vi "CRYCurve averaging real-time fft.vi"(7 "Initialize (F)":bool, 8 "Exponential averaging? (F=linear)":bool, 10 "Number of averages (no change)":i32, 11 "Input curve":dbl[](array[numeric]) format="%.2f") -> (3 "Averaged curve":dbl[](array[numeric]) format="%.2f")   [LabVIEW 2013]
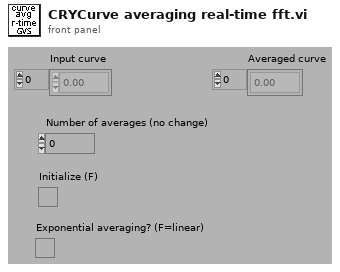
[diagram p1: front panel]
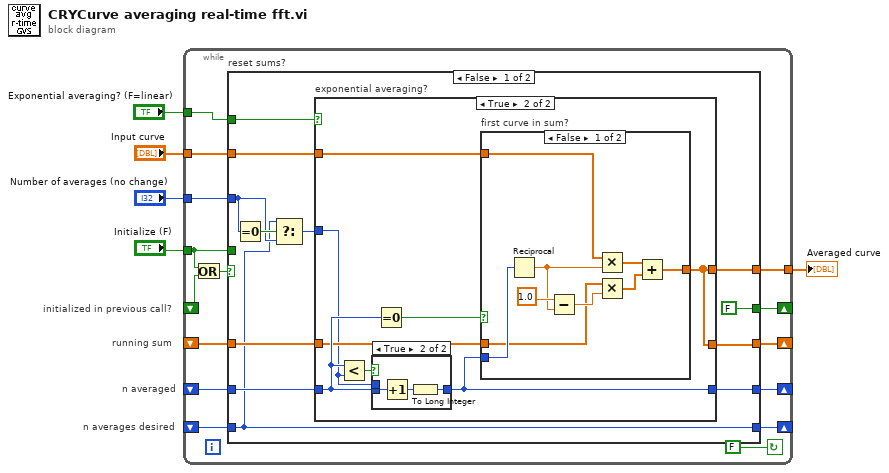
[diagram p0: block diagram]
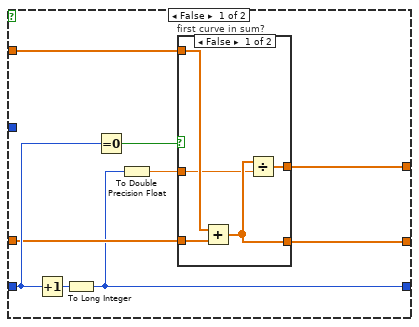
[diagram p2: hidden frame]
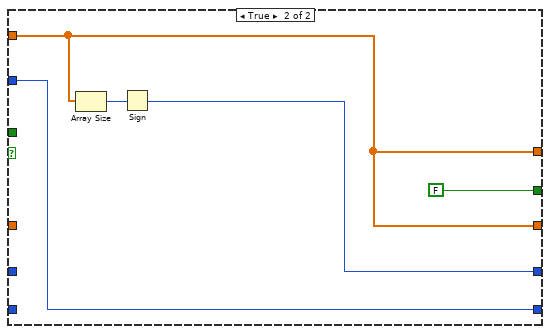
[diagram p6: hidden frame]
diagram:
  # "initialized in previous call?"
  # "n averages desired"
  # "n averaged"
  # "running sum"
  n1 = while {
    shift-left: _ -> [w8]
    shift-right: [w10] -> _
    tunnel: "Exponential averaging? (F=linear)" -> [w11]
    shift-left: _ -> [w12]
    shift-right: [w13] -> _
    tunnel: [w15] -> w2
    tunnel: "Number of averages (no change)" -> [w17]
    tunnel: "Input curve" -> [w18]
    tunnel: "Initialize (F)" -> [w9]
    shift-left: _ -> [w16]
    shift-right: [w19] -> _
    shift-left: _ -> [w14]
    shift-right: [w20] -> _
    stop <- FALSE continue-if-true
    n2 = Or(x=w9, y=w8) -> (x .or. y?=w7:bool)
    n3 = case "reset sums?" shown="False" w7 {
      tunnel: [w23 w71] -> w20
      tunnel: [w29 w70] -> w19
      tunnel: w18 -> [w31 w71]
      tunnel: w17 -> [w27 w74]
      tunnel: w16 -> [w32 _]
      tunnel: [w24 w71] -> w15
      tunnel: w14 -> [w30 _]
      tunnel: [w25 w74] -> w13
      tunnel: w12 -> [w25 _]
      tunnel: w11 -> [w22 _]
      tunnel: [FALSE ("Initialize (F)") FALSE ("Initialize (F)")] -> w10
      tunnel: w9 -> [_ _]
      frame False {
        n4 = Equal To 0?(x=w27) -> (x = 0?=w28:bool)
        n5 = Select(t=w25, s=w28, f=w27) -> (s? t:f=w26:i32)
        n6 = case "exponential averaging?" shown="True" w22 {
          tunnel: w32 -> [w40 w54]
          tunnel: w31 -> [w37 w52]
          tunnel: w30 -> [w38 w51]
          tunnel: [w34 w50] -> w29
          tunnel: [w35 w48] -> w24
          tunnel: w26 -> [_ w49]
          tunnel: [w36 w48] -> w23
          frame False {
            n7 = Increment(x=w40) -> (x+1=w41:i32)
            n8 = To Long Integer(number=w41) -> (32bit integer=w34:i32)
            n9 = Equal To 0?(x=w40) -> (x = 0?=w39:bool)
            n10 = To Double Precision Float(number=w34) -> (double precision float=w33:dbl)
            n11 = case "first curve in sum?" shown="False" w39 {
              tunnel: w38 -> [w46 _]
              tunnel: w37 -> [w45 w47]
              tunnel: [w44 w47] -> w36
              tunnel: [w43 w47] -> w35
              tunnel: w33 -> [w42 _]
              frame False {
                n12 = Add(x=w45, y=w46) -> (x+y=w44:dbl[])
                n13 = Divide(x=w44, y=w42) -> (x/y=w43:dbl[])
              }
              frame True {
              }
            }
          }
          frame True {
            n14 = Less?(x=w54, y=w49) -> (x < y?=w55:bool)
            n15 = case shown="True" w55 {
              tunnel: w54 -> [_ w69]
              tunnel: [w66 w67] -> w50
              tunnel: w49 -> [w66 _]
              frame False {
              }
              frame True {
                n16 = Increment(x=w69) -> (x+1=w68:i32)
                n17 = To Long Integer(number=w68) -> (32bit integer=w67:i32)
              }
            }
            n18 = Equal To 0?(x=w54) -> (x = 0?=w53:bool)
            n19 = case "first curve in sum?" shown="False" w53 {
              tunnel: w52 -> [w62 w65]
              tunnel: [w56 w65] -> w48
              tunnel: w51 -> [w59 _]
              tunnel: w50 -> [w64 _]
              frame False {
                n20 = Reciprocal(x=w64) -> (1/x=w61:dbl)
                n21 = Subtract(x=1.0, y=w61) -> (x-y=w60:dbl)
                n22 = Multiply(x=w62, y=w61) -> (x*y=w58:dbl[])
                n23 = Multiply(x=w59, y=w60) -> (x*y=w57:dbl[])
                n24 = Add(x=w58, y=w57) -> (x+y=w56:dbl[])
              }
              frame True {
              }
            }
          }
        }
      }
      frame True {
        n25 = Array Size(array=w71) -> (size(s)=w72:i32)
        n26 = Sign(1:w72) -> (0:w70:i32)
      }
    }
  }
  "Averaged curve" <- w2
